vi "X-_Read.vi"(0 "Address":u8, 1 "Port Name":string, 2 "COMMAND":T1, 3 "Channel Name":string, 4 "Iteration No":i32) -> (7 "Numeric Reply":dbl format="%.2f", 9 "String Reply":string, 10 "Non-Blank reply":bool)   [LabVIEW 2010]
uses:
  X-_commands.ctl
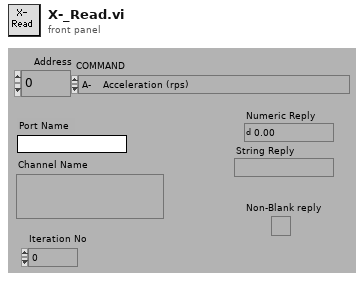
[diagram p1: front panel]
types:
  T1 = typedef "X-_commands.ctl" = enum16{"A-    Acceleration (rps)", "B-    Buffer Status", "C-    Continue", "CG-  Correction Gain", "CR-  Cariage Return", "D-    Distance (pulses)", "DB-  Dead Band (encoder steps)", "DW- Deadband Window (encoder steps)", "E-    Enable Communications", "ER-  Encoder Resolution (steps/rev)", "F-    Disable Communications", "FS-  Encoder Functions Report", "FSA- Incremental/Absolute (0/1)", "FSB- Motor/Encoder Step Mode (0/1)", "FSC- Enable/Disable Position Maint. (1/0)", "FSD- Stop/Continue on Stall (1/0)", "FSE- Activate o/p1 on Stall (1/0)", "FSF- Stop Motion on Trig3 (1/0)", "FSG- Activate o/p2 in Deadband (1/0)", "FSH- Enable Stall Detect (1/0)", "G- Go", "GH- Go Home and Zero (+/-V)", "^H- Delete ", "H- Direction Reverse/CCW/CW (0,1,2)", "IS- Input Status", "K- Kill", "L- Loop (n)", "LD- Limit DISABLE (0-none,1-CW,2-CCW,3-Both)", "LF- Line Feed", "MC- Mode Continuous", "MN- Mode Normal", "MPA- Motor Postion Absolute", "MPI- Motor Position Incremental", "MR- Motor Resolution (Drive Steps/rev)", "N- End of Loop", "O- Output (00,01,10,11)", "OS- Report Homing Setup", "OSA- NO/NC Limits (1/0)", "OSB- Back Up to Home/Edge? (0/1)", "OSC- NO/NC Home Switch (1/0)", "OSD- Enable Encoder Z for Home (0/1)", "OSH- Reference Edge for Home CW/CCW (0/1)", "PR- Report ABSOLUTE Position", "PS- Pause until Continue", "PX- Report Absolute ENCODER Position", "PZ- Zero Absolute Counter", "\"- Quote (17 ASCII +Space)", "Q- Enter/Exit Velocity Profiling (1/0)", "R- Request Indexer Status", "RA- Report Limit Switch Status", "RB- Report Loop, Pause, Shutdown, Trigger Status", "RC- Report Closed Loop Status", "RM- Velocity Streaming Rate Multiplier (000-FFF)", "RV- Report Revision Level", "S- Controlled Stop", "SN- Debounce (1-1000ms)", "SS- Report Software Switch Status", "SSA- Disable RS232 Echo (1/0)", "SSG- Clear/Save Command Buffer on Limit (0/1)", "SSH- Clear/Save Command Buffer on Stop (0/1)", "ST- Shutdown (1/0)", "SV- Servoing Setting (0,1,2,3)", "T- Time Delay (0.01-99999.99)", "TR- Wait for Trigger High/Low/Ignore (1/0/X)", "TS- Report Trigger Status", "U- Pause after Move Until Continue", "V- Velocity (0.01-50.00 revs/sec)", "W1- Report Relative Position <Signed Binary>", "W3- Report Relative Position <Hexadecimal>", "Y- Abort Loop at N", "Z-    Reset to Defaults", "#-    Disable/Set Soft Addresses (0/1-255)"}
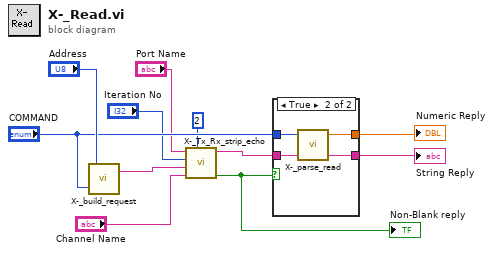
[diagram p0: block diagram]
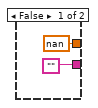
[diagram p2: hidden frame]
diagram:
  n1 = call "X-_build_request.vi"("COMMAND"="COMMAND", "Address"="Address") -> ("Write String"=w6:string)  [unwired: 1 out]
  n2 = call "X-_Tx_Rx_strip_echo.vi"("Terminate Count"=2, "Channel Name"="Channel Name", "Write String"=w6, "Iteration No"="Iteration No", "Port Name"="Port Name") -> ("Non-Blank reply"=w3:bool, "Reply"=w10:string)  [unwired: 2 out]
  "Non-Blank reply" <- w3
  n3 = case shown="True" w3 {
    tunnel: w10 -> [_ w17]
    tunnel: "COMMAND" -> [_ w16]
    tunnel: [nan ("Numeric Reply") w15] -> w8
    tunnel: ["" w14] -> w7
    frame False {
    }
    frame True {
      n4 = call "X-_parse_read.vi"("Read"=w17, "COMMAND"=w16) -> ("String Reply"=w14:string, "Numeric Reply"=w15:dbl)  [unwired: 1 in, 1 out]
    }
  }
  "String Reply" <- w7
  "Numeric Reply" <- w8
